vi "Log Data.vi"(8 "error in (no error)":errorcluster, 9 "t0":timestamp, 10 "Data in":dbl[](array[numeric]), 11 "Triggered Log in":refnum<class "Triggered Log.lvclass">) -> (0 "error out":errorcluster, 3 "Triggered Log out":refnum<class "Triggered Log.lvclass">)   [LabVIEW 2012, in "Triggered Log.lvclass"]
doc: "Processes the sampled data from <b>Data in</b> according to the current state of the triggered log.\n\nIf the triggered log is currently waiting on the start trigger, the samples are inserted into the circular pretrigger buffer, which will get flushed to disk whenever the start trigger occurs.\n\nIf the start trigger condition for the triggered log has occurred, and either the stop trigger condition has not yet occurred or the specified number of posttrigger samples has not yet been logged, then the sampled data is inserted into the data buffer. When the data buffer fills up, its contents are flushed to disk.\n\nAfter processing the sampled data, the log checks the posttrigger countdown if the stop trigger condition has occurred. When the posttrigger countdown completes, the triggered log either returns to waiting on the next start trigger or marks itself complete, depending on whether it is retriggerable.\n\nIf the triggered log is already complete, this VI does nothing with the sampled data."
uses:
  Triggered Log.lvclass
  Triggered Log.lvclass/Triggered Log.ctl
  Engine/Classes/Logs/Segmented Logs/Segmented Log/Segmented Log.lvclass/Segmented Log.ctl
  Shared/Classes/Log File Specifications/Log File Specification/Log File Specification.lvclass/Log File Specification.ctl
  Flush Buffer Data to File.vi
  Set Triggered Log State.vi
  Force Close Log File Instance.vi
  Flush Buffer Data.vi
  Engine/Classes/Logs/Segmented Logs/Segmented Log/Write Data to Log File Instance (Waveform).vi
  Engine/Classes/Logs/Segmented Logs/Segmented Log/Write Data to Log File Instance.vi
  On Triggered Log State Change.vi
  Engine/Classes/Logs/Segmented Logs/Segmented Log/Check Close File.vi
  Engine/Classes/Logs/Segmented Logs/Segmented Log/Check Open File.vi
  Engine/Classes/Logs/Segmented Logs/Segmented Log/Close Log File Instance.vi
  Engine/Classes/Logs/Segmented Logs/Segmented Log/Open Log File Instance.vi
  Engine/Classes/Logs/Segmented Logs/Segmented Log/On Segmented Log Complete.vi
  Engine/Classes/Logs/Segmented Logs/Segmented Log/On File Close.vi
  Shared/Classes/Log File Specifications/Log File Specification/Open Log File.vi
  Shared/Classes/Log File Specifications/Log File Specification/Set Path Tag.vi
  Engine/Classes/Logs/Segmented Logs/Segmented Log/On File Open.vi
  Shared/Classes/Log File Specifications/Log File Specification/Set Filename Offset.vi
  Shared/Classes/Log File Specifications/Log File Specification/Build File Path.vi
  Shared/Classes/Log File Specifications/Log File Specification/Resolve File Conflicts.vi
  Engine/Classes/Triggers/Trigger/Initialize.vi
  Engine/Classes/Triggers/Trigger/Finalize.vi
  Shared/Classes/Log File Specifications/Log File Specification/Initialize Log File.vi
  <vilib>/Utility/libraryn.llb/Check if File or Folder Exists.vi
  <vilib>/Utility/error.llb/Error Cluster From Error Code.vi
  <vilib>/Utility/libraryn.llb/Get File Extension.vi
  <vilib>/Utility/libraryn.llb/Create Directory Recursive.vi
  Engine/Classes/Logs/Log Files/Log File/Write to Log File (Waveform).vi
  Engine/Classes/Logs/Segmented Logs/Segmented Log/Segment Log File.vi
  Engine/Classes/Logs/Log Files/Log File/Close Log File.vi
  Engine/Classes/Logs/Segmented Logs/Segmented Log/Make File Read-Only.vi
  Engine/Classes/Logs/Log Files/Log File/Write to Log File.vi
  Engine/Classes/Logs/Segmented Logs/Segmented Log/Force Close Log File Instance.vi
  Engine/Classes/Logs/Log Files/Log File/Log File.lvclass
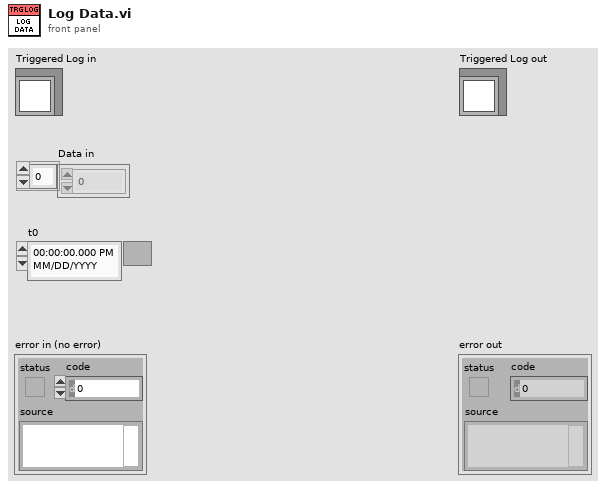
[diagram p1: front panel]
types:
  T1 = typedef "Triggered Log.lvclass/Triggered Log State.ctl" = enum16{"Waiting on Trigger", "Triggered", "Posttrigger", "Complete", "Idle", "Error"}
  T2 = typedef "Triggered Log.lvclass/Buffer Data.ctl" = cluster{"Position":i32, "Length":i32, "Max Length":i32, "Channel Count":i32, "Data":dbl[][], "t0 Array":timestamp[]}
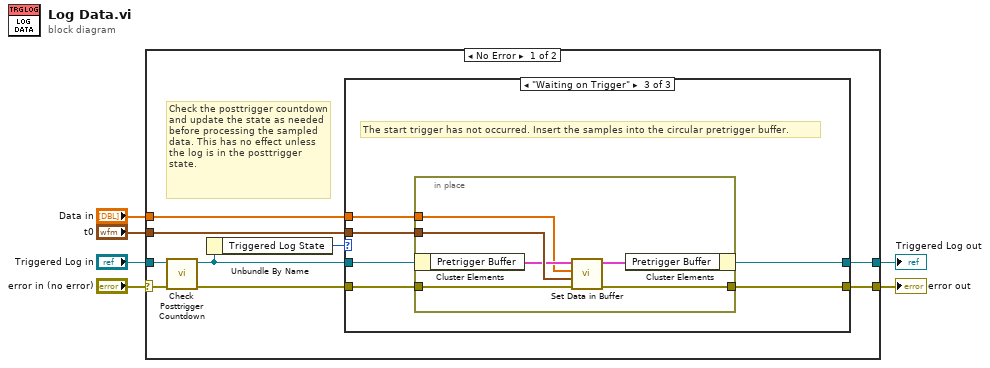
[diagram p0: block diagram]
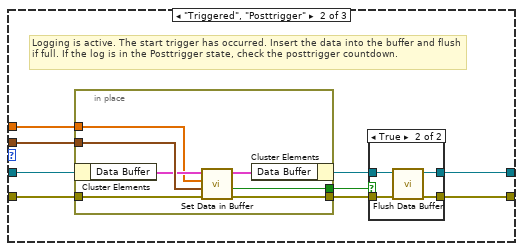
[diagram p3: hidden frame]
diagram:
  n1 = case shown="No Error" "error in (no error)" {
    selector: "error in (no error)" -> [w11 w53]
    tunnel: "Data in" -> [w15 _]
    tunnel: "Triggered Log in" -> [w9 w52]
    tunnel: [w13 w52] -> w4
    tunnel: [w12 w53] -> w3
    tunnel: "t0" -> [w7 _]
    frame No Error {
      # "Check the posttrigger countdown and update the state as needed before processing the sampled data. This has no effect unless the log is in the posttrigger state."
      n2 = call "Check Posttrigger Countdown.vi"("error in (no error)"=w11, "Triggered Log in"=w9) -> ("error out"=w10:errorcluster, "Triggered Log out"=w8:refnum<class "Triggered Log.lvclass">)  [unwired: 8 in]
      n3 = Unbundle By Name(w8) -> ("Triggered Log State"=w14:T1)
      n4 = case shown="\"Waiting on Trigger\"" w14 {
        tunnel: w15 -> [_ w26 w45]
        tunnel: [w17 w22 w43] -> w13
        tunnel: [w16 w21 w41] -> w12
        tunnel: w10 -> [w16 w20 w42]
        tunnel: w8 -> [w17 w25 w44]
        tunnel: w7 -> [_ w18 w40]
        frame "Complete".."Error" {
        }
        frame "Triggered", "Posttrigger" {
          # "Logging is active. The start trigger has occurred. Insert the data into the buffer and flush if full. If the log is in the Posttrigger state, check the posttrigger countdown."
          n5 = in-place {
            in-place-border: w26 -> [w36]
            in-place-border: [w35] -> w23
            in-place-border: w20 -> [w34]
            in-place-border: [w33] -> w19
            in-place-border: w18 -> [w39]
            n6 = in-place-cluster #1(w25) -> ("Data Buffer"=w38:T2)
            n7 = call "Set Data in Buffer.vi"("error in (no error)"=w34, "t0"=w39, "Data in"=w36, "Buffer Data in"=w38) -> ("error out"=w33:errorcluster, "Buffer Full"=w35:bool, "Buffer Data out"=w37:T2)  [unwired: 5 in]
            n8 = in-place-cluster #1("Data Buffer"=w37) -> (w24:refnum<class "Triggered Log.lvclass">)
          }
          n9 = case shown="True" w23 {
            tunnel: [w27 w32] -> w21
            tunnel: w24 -> [w28 w31]
            tunnel: [w28 w30] -> w22
            tunnel: w19 -> [w27 w29]
            frame False {
            }
            frame True {
              n10 = call "Flush Data Buffer.vi"("error in (no error)"=w29, "Triggered Log in"=w31) -> ("error out"=w32:errorcluster, "Triggered Log out"=w30:refnum<class "Triggered Log.lvclass">)  [unwired: 8 in]
            }
          }
        }
        frame "Waiting on Trigger" {
          # "The start trigger has not occurred. Insert the samples into the circular pretrigger buffer."
          n11 = in-place {
            in-place-border: w45 -> [w48]
            in-place-border: w42 -> [w47]
            in-place-border: [w46] -> w41
            in-place-border: w40 -> [w51]
            n12 = in-place-cluster #2(w44) -> ("Pretrigger Buffer"=w50:T2)
            n13 = call "Set Data in Buffer.vi"("error in (no error)"=w47, "t0"=w51, "Data in"=w48, "Buffer Data in"=w50) -> ("error out"=w46:errorcluster, "Buffer Data out"=w49:T2)  [unwired: 5 in, 1 out]
            n14 = in-place-cluster #2("Pretrigger Buffer"=w49) -> (w43:refnum<class "Triggered Log.lvclass">)
          }
        }
      }
    }
    frame Error {
    }
  }
  "error out" <- w3
  "Triggered Log out" <- w4
